vi "Test_Multi_FTP.vi"() -> ()   [LabVIEW 2009]
panel:
  out "Trj Filename":string
  in  "Ring":u16(ring) items=["Mput", "longstring", "ftpput"]
  in  "Number of Files":i32
  out "Time taken":u32
  in  "Address":string
  in  "file path (use dialog)":path=path "C:/Christian/Some_Files"
  in  "Create":bool
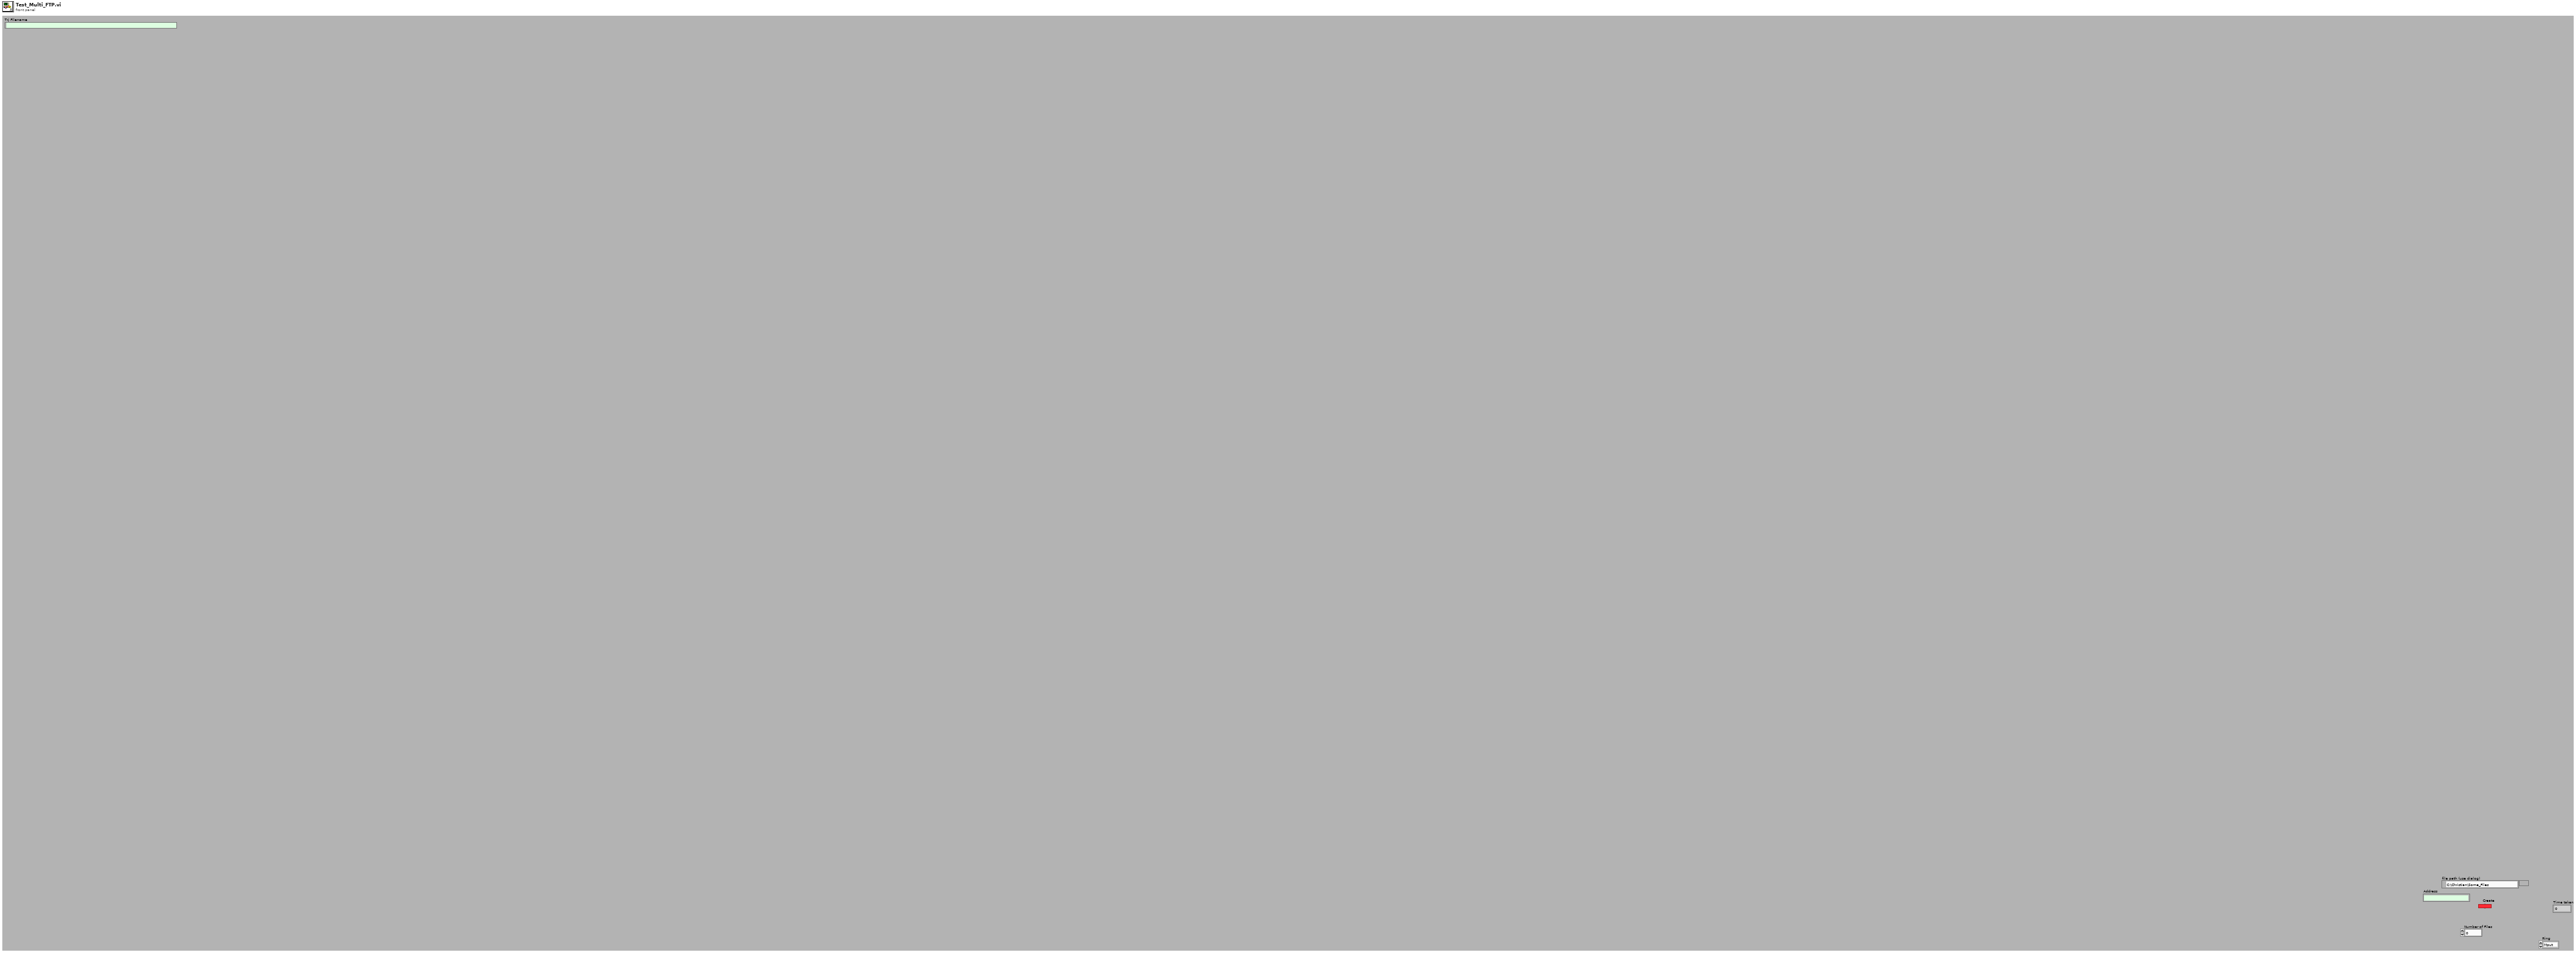
[diagram p1: front panel]
types:
  T1 = enum16{"open", "replace", "create", "open or create", "replace or create", "replace or create with confirmation"}
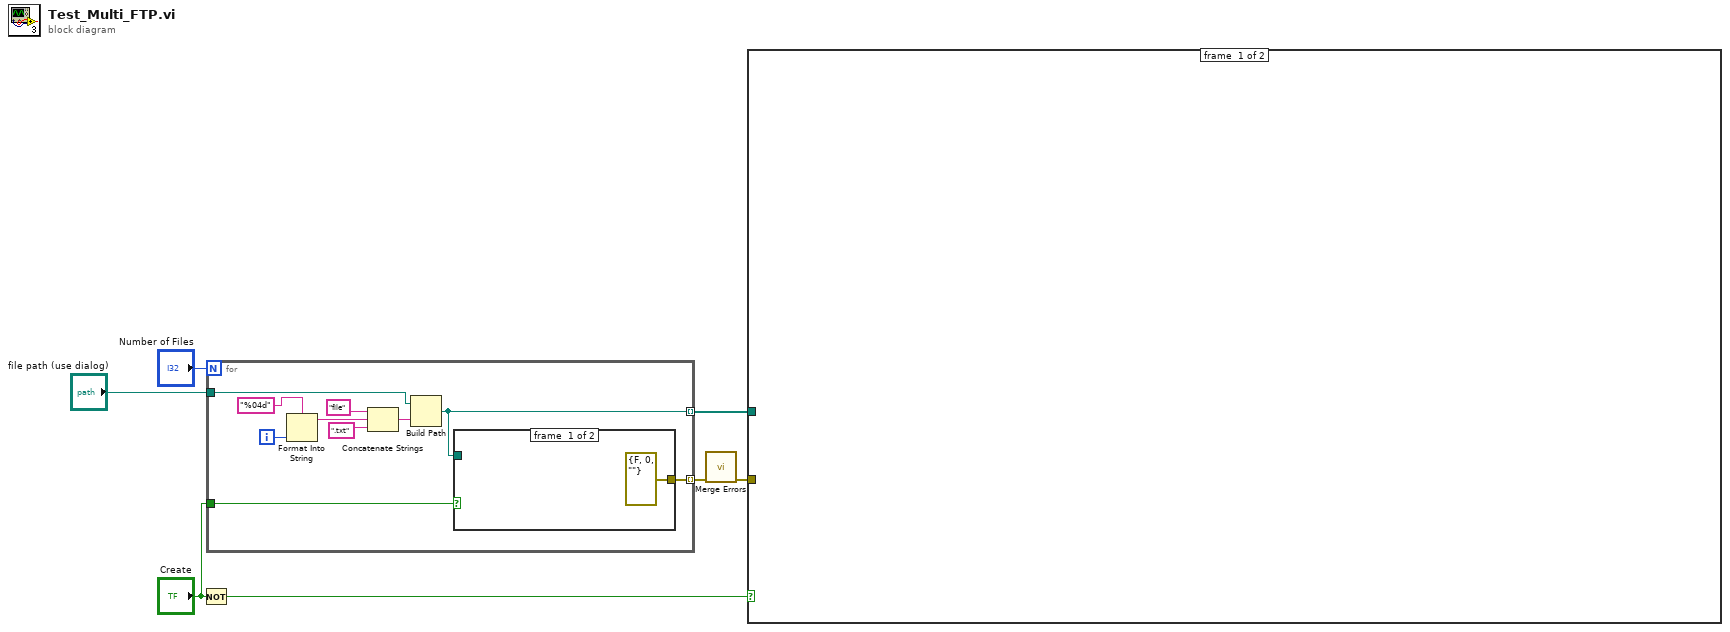
[diagram p0: block diagram]
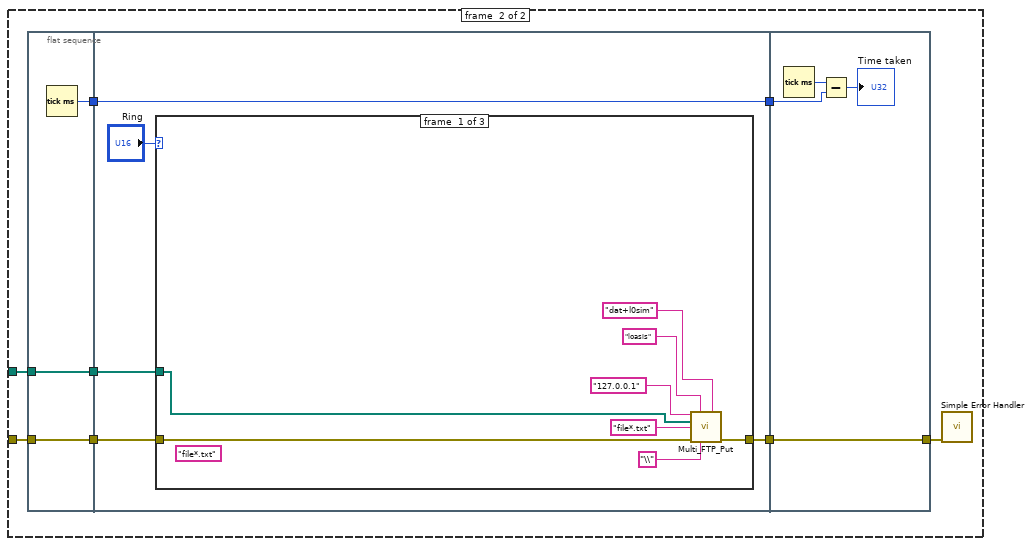
[diagram p2: hidden frame]
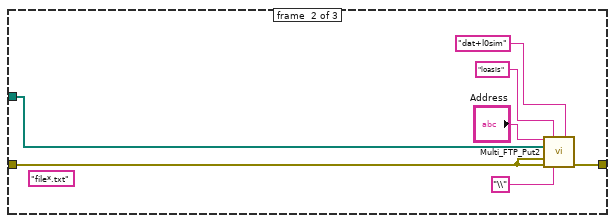
[diagram p3: hidden frame]
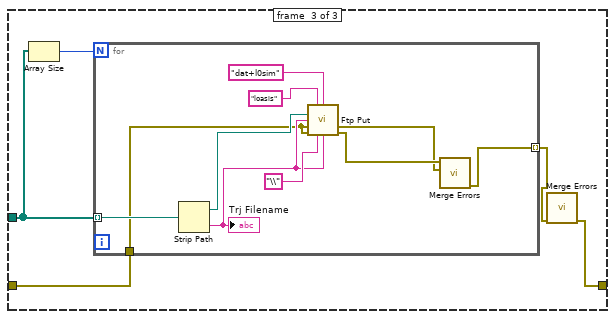
[diagram p4: hidden frame]
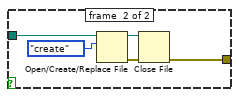
[diagram p5: hidden frame]
diagram:
  n1 = Not(x="Create") -> (.not. x?=w1:bool)
  n2 = for {
    N: "Number of Files" -> [_]
    tunnel: "file path (use dialog)" -> [w12]
    tunnel: [w9] -> w6 mode=indexing
    tunnel: [w11] -> w5 mode=indexing
    tunnel: "Create" -> [w10]
    i -> [w17]
    n3 = Format Into String(format string="%04d", w17) -> (resulting string=w16:string)  [unwired: 2 in, 1 out]
    n4 = Concatenate Strings("file" ("string"), w16, ".txt" ("string")) -> (w13:string)
    n5 = Build Path(base path=w12, name or relative path=w13) -> (appended path=w9:path)
    n6 = case shown="True" w10 {
      tunnel: w9 -> [_ w22]
      tunnel: [errorcluster {"status"=FALSE, "code"=0, "source"=""} ("error out") w19] -> w11
      frame #0 {
      }
      frame #1 {
        n7 = Open/Create/Replace File(file path (use dialog)=w22, operation (0:open)=T1."create") -> (refnum out=w21:refnum<file>, error out=w20:errorcluster)  [unwired: 4 in, 1 out]
        n8 = Close File(refnum=w21, error in=w20) -> (error out=w19:errorcluster)  [unwired: 1 out]
      }
    }
  }
  n9 = call <vilib>:"Merge Errors.vi"("error array in"=w5) -> ("error out"=w4:errorcluster)  [unwired: 6 in]
  n10 = case shown="True" w1 {
    tunnel: w6 -> [_ w28]
    tunnel: w4 -> [_ w27]
    frame #0 {
    }
    frame #1 {
      n11 = flat-sequence {
        tunnel: w28 -> [w34]
        tunnel: [w34] -> w31
        tunnel: w27 -> [w33]
        tunnel: [w33] -> w30
        tunnel: [w32] -> w29
        tunnel: w31 -> [w39]
        tunnel: w30 -> [w38]
        tunnel: [w37] -> w25
        tunnel: [w36] -> w24
        tunnel: w29 -> [w36]
        tunnel: w25 -> [w73]
        tunnel: [w73] -> w26
        tunnel: w24 -> [w71]
        frame #0 {
          n12 = Tick Count (ms)() -> (millisecond timer value=w32:u32)
        }
        frame #1 {
          n13 = case shown="1" "Ring" {
            tunnel: w39 -> [w42 w54 w59]
            tunnel: w38 -> [w40 w49 w57]
            tunnel: [w41 w48 w55] -> w37
            frame #0 {
              (unwired) "file*.txt" ("Local Files To Put (DOS Wildcards allowed)")
              n14 = call "Multi_FTP_Put.vi"("Address"="127.0.0.1" ("Address 2"), "User"="loasis", "Password"="dat+l0sim", "trj file path 2"=w42, "Local Files To Put (DOS Wildcards allowed)"="file*.txt", "error in (no error)"=w40, "Cible Directory"="\\") -> ("error out"=w41:errorcluster)  [unwired: 7 in, 1 out]
            }
            frame #1 {
              (unwired) "file*.txt" ("Local Files To Put (DOS Wildcards allowed)")
              n15 = call "Multi_FTP_Put2.vi"("Address"="Address", "User"="loasis", "Password"="dat+l0sim", "trj file path 2"=w54, "XPS error in(no error)"=w49, "error in (no error)"=w49, "Cible Directory"="\\") -> ("error out"=w48:errorcluster)  [unwired: 7 in, 1 out]
            }
            frame #2 {
              n16 = Array Size(array=w59) -> (size(s)=w58:i32)
              n17 = for {
                N: w58 -> [_]
                tunnel: w59 -> [w65] mode=indexing
                tunnel: w57 -> [w63]
                tunnel: [w60] -> w56 mode=indexing
                n18 = Strip Path(path=w65) -> (stripped path=w67:path, name=w66:string)
                "Trj Filename" <- w66
                n19 = call <userlib>:"Ftp Put.vi"("User"="loasis", "Password"="dat+l0sim", "Local Working Directory"=w67, "Local Files To Put (DOS Wildcards allowed)"=w66, "XPS error in (no error)"=w63, "error in (no error)"=w63, "Cible Directory"="\\", "Cible File Name"=w66) -> ("XPS error out"=w61:errorcluster, "error out"=w62:errorcluster)  [unwired: 6 in]
                n20 = call <vilib>:"Merge Errors.vi"("error in 2 (no error)"=w61, "error in 1 (no error)"=w62) -> ("error out"=w60:errorcluster)  [unwired: 5 in]
              }
              n21 = call <vilib>:"Merge Errors.vi"("error array in"=w56) -> ("error out"=w55:errorcluster)  [unwired: 6 in]
            }
          }
        }
        frame #2 {
          n22 = Tick Count (ms)() -> (millisecond timer value=w72:u32)
          n23 = Subtract(x=w72, y=w71) -> (x-y=→"Time taken":u32)
        }
      }
      n24 = call <vilib>:"Simple Error Handler.vi"("error in (no error)"=w26) -> ()  [unwired: 4 in, 5 out]
    }
  }
